vi "Celda solar automatizada.vi"() -> ()   [LabVIEW 2014]
uses:
  <vilib>/imath/engines/lvmath2/RunTimeEngine/ArithmeticOperatorToken/NIMS_ArithmeticOperator_power(S).vi
  <instcachedir>/0/NIMS_ArithmeticOperator_power(S)_CAFE680B12A64A3A8F5E28A20C679B7D.lvgen/NIMS_ArithmeticOperator_power(S)_CAFE680B12A64A3A8F5E28A20C679B7D_014.vi
  <vilib>/imathl/engines/lvmath/Functions/Error Handling/Create Error.vi
  <vilib>/imath/engines/lvmath2/RunTimeEngine/CommandStatement/MC_CommandStatement_break.vi
  <vilib>/imath/engines/lvmath2/RunTimeEngine/RangeToken/NIMS_Range_R2 - Integer.vi
  <instcachedir>/0/NIMS_Range_R2 - Integer_2D1304BAF97744E0A293025746CBADFC.lvgen/NIMS_Range_R2 - Integer_2D1304BAF97744E0A293025746CBADFC_000.vi
  <vilib>/imath/engines/lvmath2/RunTimeEngine/IndexReplace/NIMS V(S)=S.vi
  <instcachedir>/0/NIMS V(S)=S_2D52C4EC15D8415E870AEE69FB516CCA.lvgen/NIMS V(S)=S_2D52C4EC15D8415E870AEE69FB516CCA_001.vi
  <instcachedir>/0/NIMS V(S)=S_2D52C4EC15D8415E870AEE69FB516CCA.lvgen/NIMS V(S)=S_2D52C4EC15D8415E870AEE69FB516CCA_000.vi
  <vilib>/imath/engines/lvmath2/RunTimeEngine/CommandStatement/NIMS_CommandStatement_MaskErr.vi
  <vilib>/imath/engines/lvmath2/RunTimeEngine/NodeEndStatement/NIMS_NodeEndStatement_Output.vi
  <instcachedir>/0/NIMS_NodeEndStatement_Output_53EC0D466D134D7ABD903AC30B43404B.lvgen/NIMS_NodeEndStatement_Output_53EC0D466D134D7ABD903AC30B43404B_000.vi
  <instcachedir>/0/NIMS_NodeEndStatement_Output_53EC0D466D134D7ABD903AC30B43404B.lvgen/NIMS_NodeEndStatement_Output_53EC0D466D134D7ABD903AC30B43404B_005.vi
  <vilib>/imath/engines/lvmath2/RunTimeEngine/ErrorHandling/NIMS_Finalize Error.vi
panel:
  out "x*y":cdb[](array[numeric])
  in  "Tab Control":enum32{"Page 2"}(tab)
  in  "Resistencia de carga":dbl
  out "Curva de Potencia":cluster{dbl[], dbl[]}(graph)
  in  "Temperatura":dbl
  in  "Irradiancia":dbl caption="Radiaccion" step=0.05
  in  "?":enum32{"Predeterminado", "Avanzado"}(tab)
  out "Factor de calidad":dbl=1.2
  out "T1":dbl=1.2
  out "Voc T1":dbl=1.2
  out "Isc T1":dbl=1.2
  out "T2":dbl=1.2
  out "Voc T2":dbl=1.2
  out "Isc T2":dbl=1.2
  in  "Principales Marcas":u16(ring) items=["Solarex MSX60", "Jinko Solar Perc 60-JKM300M-60", "Suntech STP275S-20", "Trina Solar TSM-250PD05", "Canadian Solar CS6X-305P", "JA Solar JAM6 PR mono 60", "Hanwha Q.Peak-G4.1", "Sharp ND-F2Q235", "Yingli YGE Serie YL275P-29b", "SolarWorld SW290", "Kyocera KD265GX-LFB\""]
  out "Vg":dbl=1.2
  out "Celdas en serie":dbl
  in  "Factor de calidad":dbl
  in  "Vg":dbl
  in  "T1":dbl
  in  "Voc T1":dbl
  in  "Isc T1":dbl
  in  "T2":dbl
  in  "Voc T2":dbl
  in  "Isc T2":dbl
  in  "Celdas en series":dbl
  out "Curva Caracteristica I-V":cluster{"Vao":dbl[], "Iao":dbl[]}[](graph)
  out "?":string
  in  "stop":bool
  in  "Paneles en serie":dbl min=1.0
  in  "Paneles en paralelo":dbl min=1.0
  out "modelo":string
  out "String":string
  out "Numeric":i32
  out "Ia":cdb[](array[numeric])
  # "Curva 1: curva característica del panel solar\n\nCurva 2: recta de carga"
  # "Curva 1: curva de potencia del panel solar"
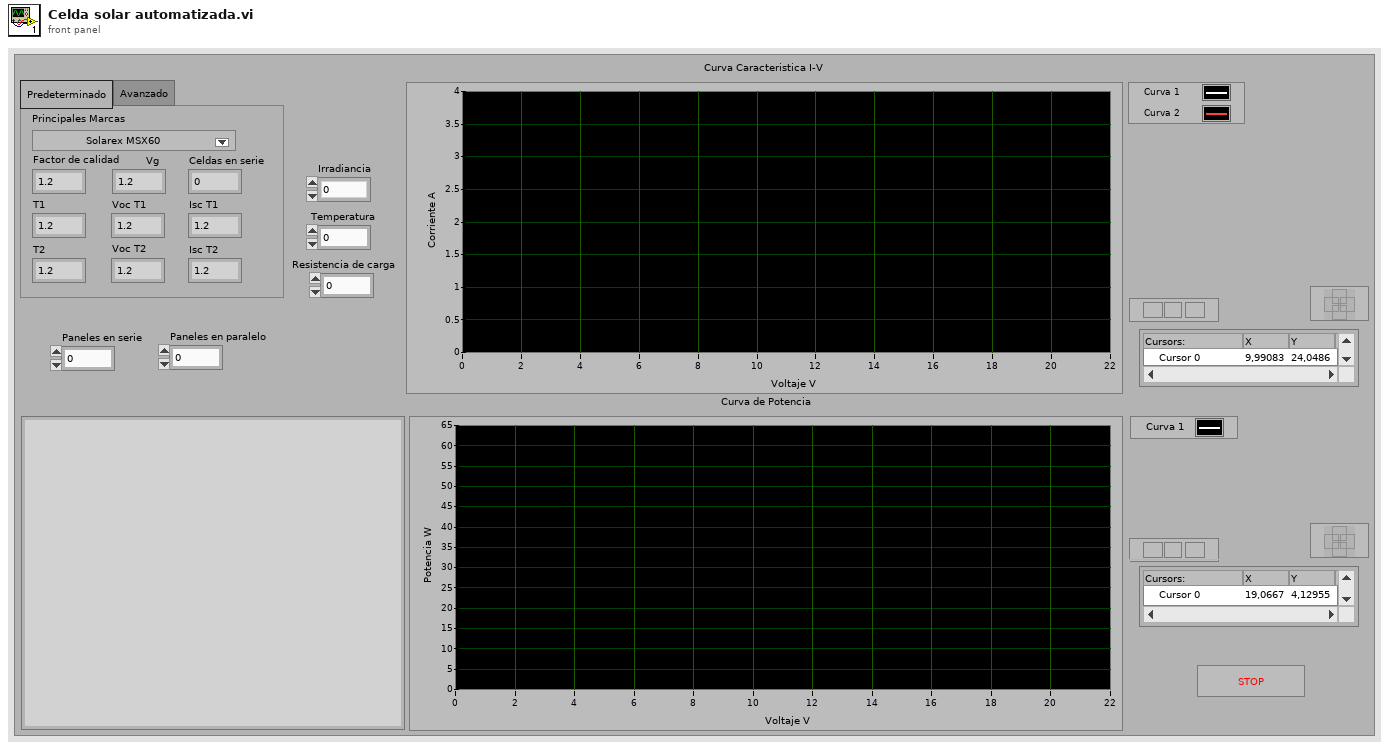
[diagram p1: front panel]
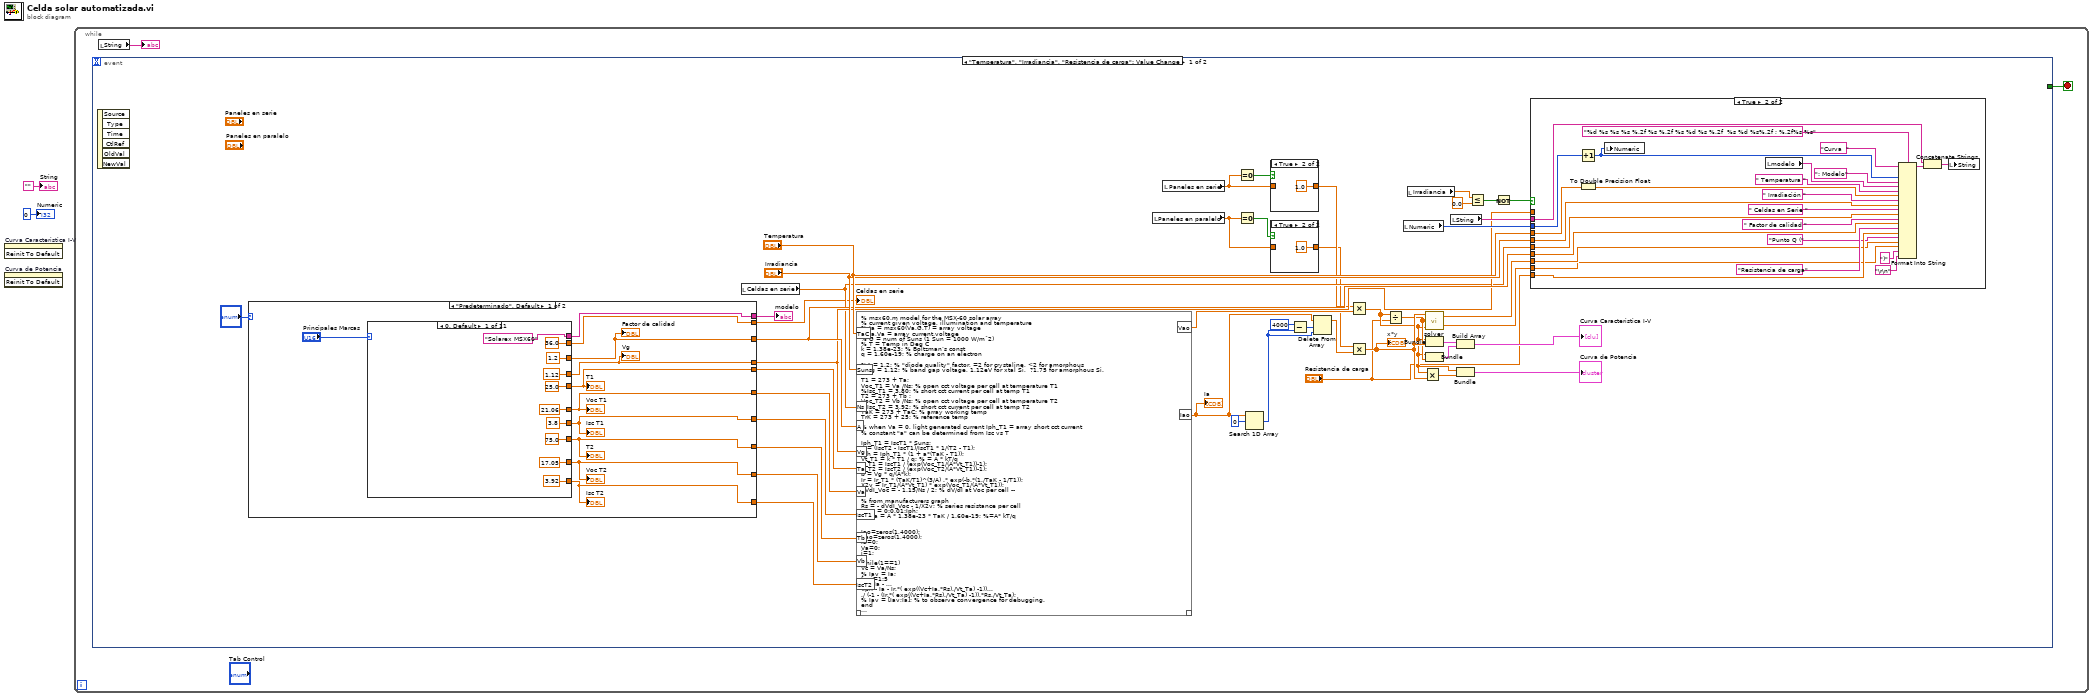
[diagram p0: block diagram]
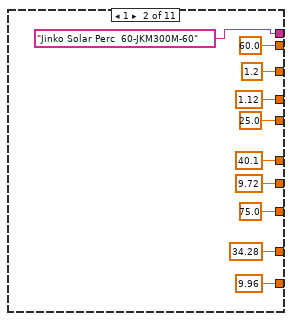
[diagram p4: hidden frame]
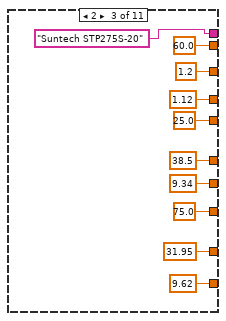
[diagram p5: hidden frame]
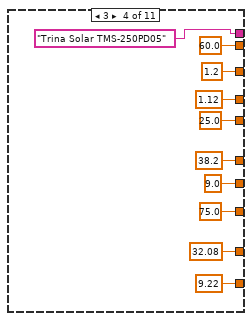
[diagram p6: hidden frame]
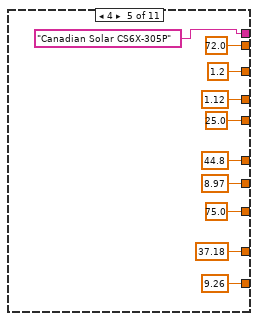
[diagram p7: hidden frame]
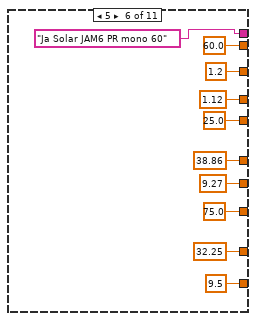
[diagram p8: hidden frame]
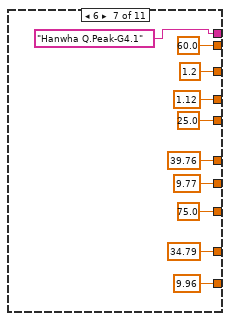
[diagram p9: hidden frame]
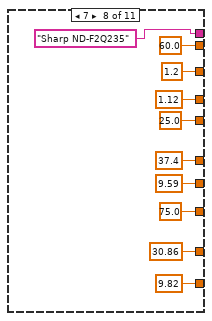
[diagram p10: hidden frame]
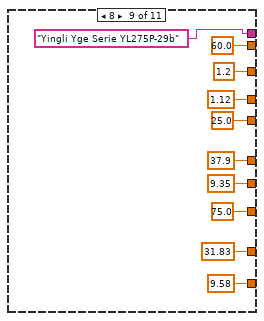
[diagram p11: hidden frame]
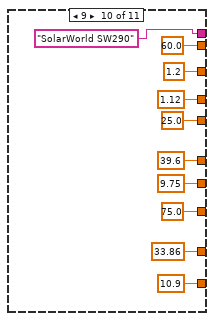
[diagram p12: hidden frame]
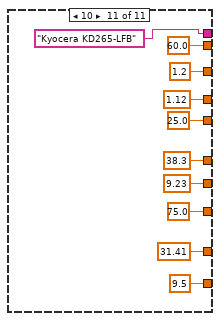
[diagram p13: hidden frame]
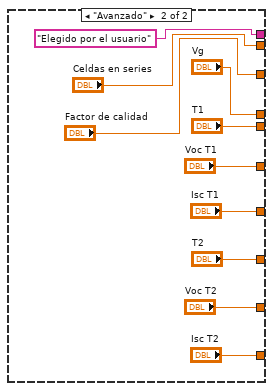
[diagram p14: hidden frame]
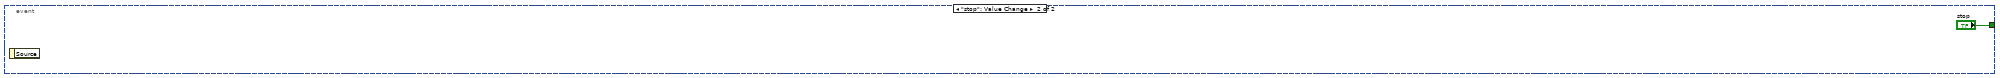
[diagram p16: hidden frame]
diagram:
  n1 = invoke on="Curva Caracteristica I-V" class="XYGraph (strict)" method="Reinit To Default"() -> ()  [unwired: 3 in, 3 out]
  n2 = invoke on="Curva de Potencia" class="XYGraph (strict)" method="Reinit To Default"() -> ()  [unwired: 3 in, 3 out]
  n3 = while {
    stop <- w4 stop-if-true
    n4 = event shown="[0] \"Temperatura\", \"Irradiancia\", \"Resistencia de carga\": Value Change" {
      selector: _ -> [_ _]
      dyn-events: _ -> [_ _]
      timeout: _ -> [_ _]
      tunnel: [_ "stop"] -> w4
      event "Temperatura", "Irradiancia", "Resistencia de carga": Value Change {
        n5 = event-data() -> ()  [unwired: 1 in, 6 out]
        n6 = case shown="\"Predeterminado\", Default" "?" {
          tunnel: [w62 "Factor de calidad"] -> w38
          tunnel: [w61 "Vg"] -> w37
          tunnel: [w60 "T1"] -> w32
          tunnel: [w59 "Voc T1"] -> w36
          tunnel: [w58 "Isc T1"] -> w31
          tunnel: [w57 "T2"] -> w35
          tunnel: [w56 "Voc T2"] -> w34
          tunnel: [w55 "Isc T2"] -> w33
          tunnel: [w54 "Celdas en series"] -> w28
          tunnel: [w53 "Elegido por el usuario"] -> w27
          frame "Predeterminado", Default {
            n7 = case shown="0, Default" "Principales Marcas" {
              tunnel: [1.2 1.2 1.2 1.2 1.2 1.2 1.2 1.2 1.2 1.2 1.2] -> w62
              tunnel: [1.12 1.12 1.12 1.12 1.12 1.12 1.12 1.12 1.12 1.12 1.12] -> w61
              tunnel: [25.0 25.0 25.0 25.0 25.0 25.0 25.0 25.0 25.0 25.0 25.0] -> w60
              tunnel: [21.06 40.1 38.5 38.2 44.8 38.86 39.76 37.4 37.9 39.6 38.3] -> w59
              tunnel: [3.8 9.72 9.34 9.0 8.97 9.27 9.77 9.59 9.35 9.75 9.23] -> w58
              tunnel: [75.0 75.0 75.0 75.0 75.0 75.0 75.0 75.0 75.0 75.0 75.0] -> w57
              tunnel: [17.05 34.28 31.95 32.08 37.18 32.25 34.79 30.86 31.83 33.86 31.41] -> w56
              tunnel: [3.92 9.96 9.62 9.22 9.26 9.5 9.96 9.82 9.58 10.9 9.5] -> w55
              tunnel: [36.0 60.0 60.0 60.0 72.0 60.0 60.0 60.0 60.0 60.0 60.0] -> w54
              tunnel: ["Solarex MSX60" "Jinko Solar Perc  60-JKM300M-60" "Suntech STP275S-20" "Trina Solar TMS-250PD05" "Canadian Solar CS6X-305P" "Ja Solar JAM6 PR mono 60" "Hanwha Q.Peak-G4.1" "Sharp ND-F2Q235" "Yingli Yge Serie YL275P-29b" "SolarWorld SW290" "Kyocera KD265-LFB"] -> w53
              frame 0, Default {
              }
              frame 1 {
              }
              frame 2 {
              }
              frame 3 {
              }
              frame 4 {
              }
              frame 5 {
              }
              frame 6 {
              }
              frame 7 {
              }
              frame 8 {
              }
              frame 9 {
              }
              frame 10 {
              }
            }
            "Factor de calidad" <- w62
            "Vg" <- w61
            "T1" <- w60
            "Voc T1" <- w59
            "Isc T1" <- w58
            "T2" <- w57
            "Voc T2" <- w56
            "Isc T2" <- w55
          }
          frame "Avanzado" {
          }
        }
        "Celdas en serie" <- w28
        "modelo" <- w27
        n8 = local read "Celdas en serie"() -> (w29:dbl)
        n9 = mathscript code="% msx60.m model for the MSX-60 solar array\n% current given voltage, illumination and temperature\n% Ia = msx60(Va,G,T) = array voltage\n% Ia,Va = array current,voltage\n% G = num of Suns (1 Sun = 1000 W/mˆ2)\n% T = Temp in Deg C\nk = 1.38e-23; % Boltzman’s const\nq = 1.60e-19; % charge on an electron\n\n%A = 1.2; % \"diode quality\" factor, =2 for crystaline, <2 for amorphous\n%Vg = 1.12; % band gap voltage, 1.12eV for xtal Si,  ?1.75 for amorphous Si.\n\nT1 = 273 + Ta;\nVoc_T1 = Va /Ns; % open cct voltage per cell at temperature T1\n%Isc_T1 = 3.80; % short cct current per cell at temp T1\nT2 = 273 + Tb ;\nVoc_T2 = Vb /Ns; % open cct voltage per cell at temperature T2\n%Isc_T2 = 3.92; % short cct current per cell at temp T2\nTaK = 273 + TaC; % array working temp\nTrK = 273 + 25; % reference temp\n\n% when Va = 0, light generated current Iph_T1 = array short cct current\n% constant \"a\" can be determined from Isc vs T\n\nIph_T1 = IscT1 * Suns;\na = (IscT2 - IscT1)/IscT1 * 1/(T2 - T1);\nIph = Iph_T1 * (1 + a*(TaK - T1));\nVt_T1 = k * T1 / q; % = A * kT/q\nIr_T1 = IscT1 / (exp(Voc_T1/(A*Vt_T1))-1);\nIr_T2 = IscT2 / (exp(Voc_T2/(A*Vt_T1))-1);\nb = Vg * q/(A*k);\nIr = Ir_T1 * (TaK/T1)^(3/A) .* exp(-b.*(1./TaK - 1/T1));\nX2v = Ir_T1/(A*Vt_T1) * exp(Voc_T1/(A*Vt_T1));\ndVdI_Voc = - 1.15/Ns / 2; % dV/dI at Voc per cell --\n\n% from manufacturers graph\nRs = - dVdI_Voc - 1/X2v; % series resistance per cell\n% Ia = 0:0.01:Iph;\nVt_Ta = A * 1.38e-23 * TaK / 1.60e-19; %=A* kT/q\n\n\nIao=zeros(1,4000);\nVao=zeros(1,4000);\nIa=0;\nVa=0;\ni=1;\n\nwhile(1==1)\nVc = Va/Ns;\n% Iav = Ia;\nfor j=1:5\nIa= Ia - ...\n(Iph - Ia - Ir.*( exp((Vc+Ia.*Rs)./Vt_Ta) -1))...\n./ (-1 - (Ir.*( exp((Vc+Ia.*Rs)./Vt_Ta) -1)).*Rs./Vt_Ta);\n% Iav = [Iav;Ia]; % to observe convergence for debugging.\nend\n\nif(Ia<=0) break\nend\n\nIao(i)=Ia;\nVao(i)=Va;\n\ni=i+1;\nVa=Va+1/100;\n\nend"("TaC"="Temperatura", "Suns"="Irradiancia", "Ns"=w29, "Vg"=w37, "A"=w38, "Ta"=w32, "Va"=w36, "IscT1"=w31, "Tb"=w35, "Vb"=w34, "IscT2"=w33) -> ("Iao"=w26:cdb[], "Vao"=w24:dbl[])  [unwired: 1 in, 1 out]
        "Ia" <- w26
        n10 = local read "Paneles en paralelo"() -> (w18:dbl)
        n11 = local read "Paneles en serie"() -> (w21:dbl)
        n12 = Equal To 0?(x=w21) -> (x = 0?=w23:bool)
        n13 = Equal To 0?(x=w18) -> (x = 0?=w20:bool)
        n14 = Search 1D Array(1D array=w26, element=0) -> (index of element=w45:i32)  [unwired: 1 in]
        n15 = case shown="True" w23 {
          tunnel: [w51 1.0] -> w22
          tunnel: w21 -> [w51 _]
          frame False {
          }
          frame True {
          }
        }
        n16 = case shown="True" w20 {
          tunnel: [w49 1.0] -> w19
          tunnel: w18 -> [w49 _]
          frame False {
          }
          frame True {
          }
        }
        n17 = Subtract(x=4000, y=w45) -> (x-y=w46:i32)
        n18 = Delete From Array(array=w26, length=w46, index=w45) -> (array with subset deleted=w25:cdb[])  [unwired: 1 out]
        n19 = Multiply(x=w22, y=w24) -> (x*y=w14:dbl[])
        n20 = Multiply(x=w19, y=w25) -> (x*y=w16:cdb[])
        "x*y" <- w16
        n21 = Divide(x=w14, y="Resistencia de carga") -> (x/y=w15:dbl[])
        n22 = local read "Numeric"() -> (w42:i32)
        n23 = local read "Irradiancia"() -> (w7:dbl)
        n24 = Multiply(x=w14, y=w16) -> (x*y=w17:cdb[])
        n25 = call "solver.vi"("Voltaje"=w14, "Ec 2"=w15, "Ec 1"=w16) -> ("y"=w11:dbl, "x"=w12:dbl)
        n26 = Bundle(w14, w16) -> (w44:cluster{dbl[], cdb[]})  [unwired: 1 in]
        n27 = Bundle(w14, w15) -> (w13:cluster{dbl[], dbl[]})  [unwired: 1 in]
        n28 = local read "String"() -> (w41:string)
        n29 = Build Array(w44, w13) -> (→"Curva Caracteristica I-V":cluster{dbl[], cdb[]}[])
        n30 = Bundle(w14, w17) -> (→"Curva de Potencia":cluster{dbl[], cdb[]})  [unwired: 1 in]
        n31 = Less Or Equal?(x=w7, y=0.0) -> (x <= y?=w6:bool)
        n32 = Not(x=w6) -> (.not. x?=w5:bool)
        n33 = case shown="True" w5 {
          tunnel: w42 -> [_ w727]
          tunnel: w41 -> [_ w723]
          tunnel: "Temperatura" -> [_ w710]
          tunnel: "Irradiancia" -> [_ w719]
          tunnel: w29 -> [_ w717]
          tunnel: w38 -> [_ w715]
          tunnel: w37 -> [_ _]
          tunnel: w12 -> [_ w706]
          tunnel: w11 -> [_ w705]
          tunnel: "Resistencia de carga" -> [_ w708]
          frame False {
          }
          frame True {
            n34 = Increment(x=w727) -> (x+1=w724:i32)
            n35 = To Double Precision Float(number=w710) -> (double precision float=w711:dbl)
            n36 = local write "Numeric"(w724) -> ()
            n37 = local read "modelo"() -> (w712:string)
            n38 = Format Into String(format string="%d %s %s %s %.2f %s %.2f %s %d %s %.2f  %s %d %s%.2f ; %.2f%s %s", initial string="Curva  ", w724, ": Modelo", w712, " Temperatura ", w711, " Irradiación ", w719, " Celdas en Serie ", w717, " Factor de calidad ", w715, "Resistencia de carga", w708, "Punto Q (", w706, w705, ")", "\r\n") -> (resulting string=w725:string)  [unwired: 1 in, 1 out]
            n39 = Concatenate Strings(w723, w725) -> (w722:string)
            n40 = local write "String"(w722) -> ()
          }
        }
      }
      event "stop": Value Change {
        n41 = event-data() -> ()  [unwired: 1 in, 1 out]
      }
    }
    n42 = local read "String"() -> (→"?":string)
  }
  "Numeric" <- 0
  "String" <- ""
